vi "Get_GPIB_Resouces.vi"(8 "error in (no error)":errorcluster) -> (0 "error out":errorcluster, 2 "Get_GPIB_Resources":string[](array[string]), 3 "Reference out":refnum<k24>)   [LabVIEW 2017]
uses:
  D:/test/FULLband-sts/Fullband_Sample/DLL/InstrumentDLL.dll
  DLL/InstrumentDLL.dll
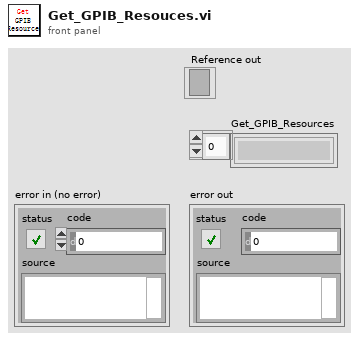
[diagram p1: front panel]
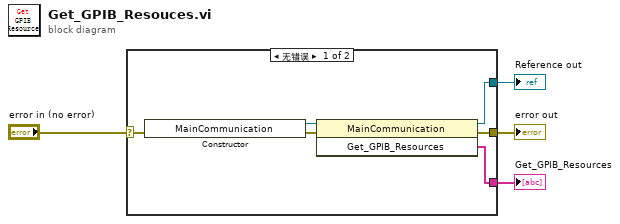
[diagram p0: block diagram]
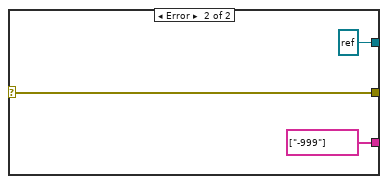
[diagram p2: hidden frame]
diagram:
  n1 = case shown="无错误" "error in (no error)" {
    selector: "error in (no error)" -> [w5 w13]
    tunnel: [w10 string[] ["-999"] ("Get_GPIB_Resources")] -> w4
    tunnel: [w7 refnum<k24> refnum ("new reference")] -> w3
    tunnel: [w6 w13] -> w2
    frame No Error {
      n2 = constructor class="MainCommunication"(error in=w5) -> (reference out=w9:refnum<k24>, error out=w8:errorcluster)  [unwired: 2 in, 1 out]
      n3 = invoke class="MainCommunication" method="Get_GPIB_Resources"(reference=w9, error in=w8) -> (reference out=w7:refnum<k24>, error out=w6:errorcluster, "Get_GPIB_Resources"=w10:string[])  [unwired: 1 in]
    }
    frame Error {
    }
  }
  "Get_GPIB_Resources" <- w4
  "Reference out" <- w3
  "error out" <- w2
